vi "启动整机测试 (子VI).vi"() -> (0 "error out":T1={"status"=FALSE, "代码"=4, "source"=""} caption="错误输出" {"代码" items=["执行成功"=1, "执行失败，但不知道原因"=2, "命令请求条件错误"=3, "通讯超时"=4, "系统繁忙不能执行"=5, "系统故障"=6, "没有数据"=100]})   [LabVIEW 2016, in "MB SLAVE.lvlib"]
uses:
  MB SLAVE.lvlib
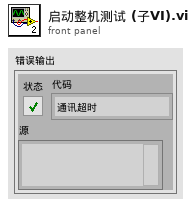
[diagram p1: front panel]
types:
  T1 = cluster{"status":bool, "代码":u16, "source":string}
  T2 = typedef "系统交互.ctl" = cluster{"运行模式":enum16{"维护模式", "常规模式", "应急模式", "质控模式", "性能测试"}, "运行间隔":i16, "流程运行中":bool, "自动运行启动参数":T3, "SYSTEM Interface.总磷总氮类型":enum16{"单模块", "总磷总氮二合一模块", "氨氮总磷二合一模块"}, "多参数运行间隔":i16, "配水时间":dbl, "沉淀时间":dbl, "清洗时间":dbl, "关键参数改变":bool, "温度告警":bool, "湿度告警":bool, "烟感告警":bool, "水浸告警":bool, "开门告警":bool, "SystemTask":enum16{"停机", "待机", "调试", "水样采集", "沉沙", "进样", "仪表测试分析", "反吹", "清洗", "除藻"}, "PumpState":enum16{"--", "只用泵1", "只用泵2", "双泵交替"}, "除藻选择":enum16{"不开除藻", "开除藻"}, "报警信息":enum16{"无报警", "断电报警", "采样管理欠压（源水泵故障）", "进样管路欠压（进样泵/增加泵故障）"}, "软件升级":bool, "固件升级":enum16{"无", "CODMn", "氨氮", "总磷", "总氮", "CODCr"}, "数据传输软件升级":bool, "数采仪软件版本":string}
  T3 = typedef "启动参数.ctl" = cluster{"氨氮":bool, "总磷":bool, "总氮":bool, "多参数":bool, "CODmn":bool, "CODCr":bool, "氟化物":bool, "超标留样":bool, "重金属":bool, "挥发酚":bool}
  T4 = typedef "参数.ctl" = cluster{"测试模式":enum16{"水样测试", "平行样测试", "集成干预测试", "加标回收"}, "参数启用":T3}
  T5 = cluster{"测试模式":enum16{"水样测试", "平行样测试", "集成干预测试", "加标回收"}, "自动运行启动参数":T3}
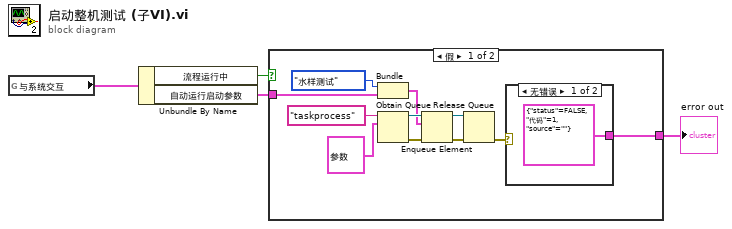
[diagram p0: block diagram]
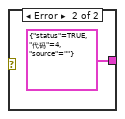
[diagram p2: hidden frame]
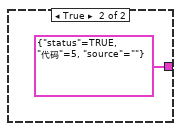
[diagram p3: hidden frame]
diagram:
  n1 = global read "modbus slave全局.vi" "与系统交互"() -> (w3:T2)
  n2 = Unbundle By Name(w3) -> ("流程运行中"=w2:bool, "自动运行启动参数"=w1:T3)
  n3 = case shown="假" w2 {
    tunnel: [w15 T1 {"status"=TRUE, "代码"=5, "source"=""} ("error out")] -> w4
    tunnel: w1 -> [w7 _]
    frame False {
      n4 = Bundle("测试模式"=enum16{"水样测试", "平行样测试", "集成干预测试", "加标回收"}."水样测试", "自动运行启动参数"=w7) -> (w5:T5)  [unwired: 1 in]
      n5 = Obtain Queue(name (unnamed)="taskprocess" ("名称（未命名）"), element data type=T4 {"测试模式"=enum."水样测试", "参数启用"={"氨氮"=FALSE, "总磷"=FALSE, "总氮"=FALSE, "多参数"=FALSE, "CODmn"=FALSE, "CODCr"=FALSE, "氟化物"=FALSE, "超标留样"=FALSE, "重金属"=FALSE, "挥发酚"=FALSE}} ("参数")) -> (queue out=w13:refnum<queue>, error out=w12:errorcluster)  [unwired: 3 in, 1 out]
      n6 = Enqueue Element(queue=w13, element=w5, error in (no error)=w12) -> (queue out=w10:refnum<queue>, error out=w11:errorcluster)  [unwired: 1 in, 1 out]
      n7 = Release Queue(queue=w10, error in (no error)=w11) -> (error out=w9:errorcluster)  [unwired: 1 in, 2 out]
      n8 = case shown="无错误" w9 {
        tunnel: [T1 {"status"=FALSE, "代码"=1, "source"=""} ("error out") T1 {"status"=TRUE, "代码"=4, "source"=""} ("error out")] -> w15
        frame No Error {
        }
        frame Error {
        }
      }
    }
    frame True {
    }
  }
  "error out" <- w4
